vi "ReadVRMLog.vi"() -> (0 "time stamp":timestamp, 1 "X Field":dbl)   [LabVIEW 2013]
uses:
  <vilib>/Utility/file.llb/Read From Spreadsheet File (DBL).vi
  <vilib>/Utility/file.llb/Write To Spreadsheet File (DBL).vi
panel:
  in  "Tab Control":enum32{"Retrieved Log", "Storage"}(tab)
  out "XY Graph":cluster{timestamp[], dbl[]}(graph)
  out "XY Graph 2":cluster{"all rows":dbl[], "all rows":dbl[]}(graph)
  out "Set Points":dbl[][](graph)
  out "Magnet":dbl[][](graph)
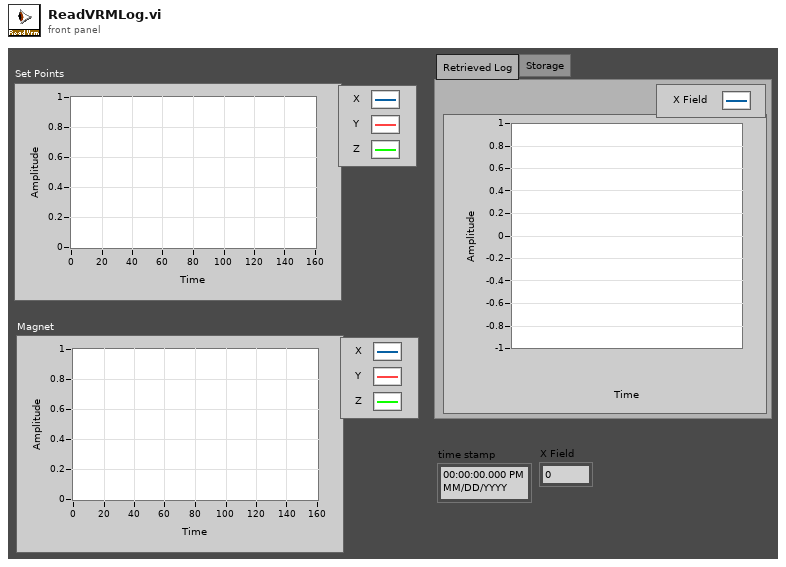
[diagram p1: front panel]
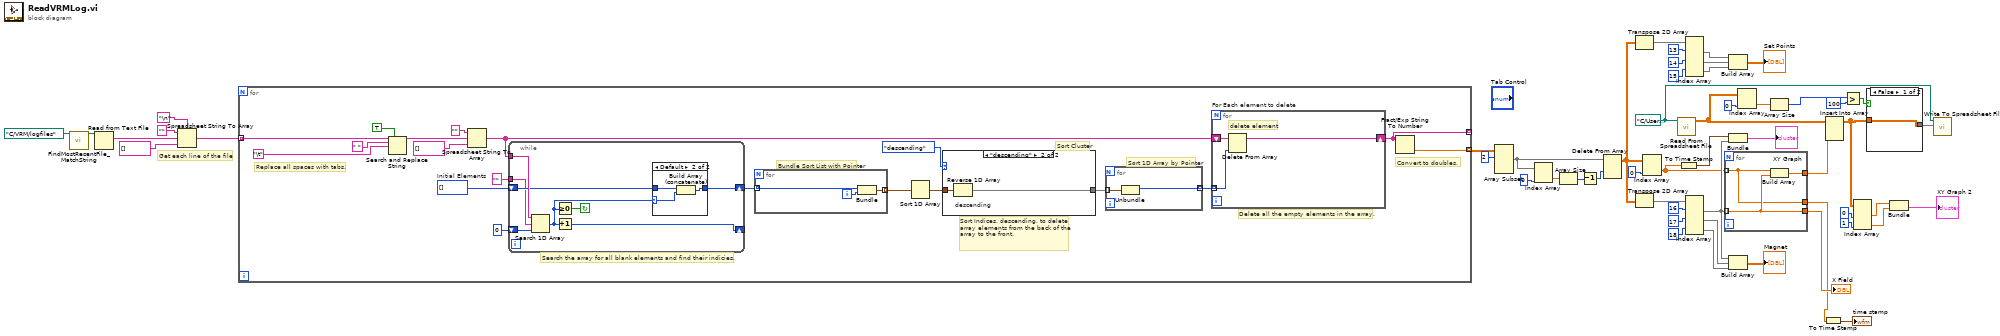
[diagram p0: block diagram]
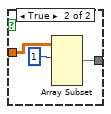
[diagram p2: hidden frame]
diagram:
  w23 = path "C:/Users/Voodoo/Desktop/Yun-Yi Pai/20140711 Log 2/Storage.txt" ("file path (dialog if empty)")
  # "Get each line of the file"
  n1 = call "FindMostRecentFile_MatchString.vi"("Folder Path In"=path "C:/VRM/logfiles") -> ("File Path Out"=w11:path)  [unwired: 9 in, 1 out]
  n2 = Read from Text File(file (use dialog)=w11) -> (text=w53:string)  [unwired: 1 in, 5 out]
  n3 = Spreadsheet String To Array(delimiter (Tab)="\n", format string="", spreadsheet string=w53, array type (2D Dbl)=string[] []) -> (array=w49:string[])
  n4 = for {
    tunnel: w49 -> [w72] mode=indexing
    tunnel: [w54] -> _ mode=indexing
    tunnel: [w55] -> w19 mode=indexing
    w64 = i32[] []  # Initial Elements
    # "Convert to doubles."
    # "Delete all the empty elements in the array."
    # "Search the array for all blank elements and find their indicies."
    # "Replace all spaces with tabs."
    # "Sort 1D Array by Pointer"
    # "Sort Cluster"
    # "Bundle Sort List with Pointer"
    # "Sort Indices, descending, to delete array elements from the back of the array to the front."
    n5 = Search and Replace String(replace all?=TRUE ("replace all? (F)"), input string=w72, search string=" ", replace string="\t") -> (result string=w67:string)  [unwired: 1 in, 6 out]
    n6 = Spreadsheet String To Array(format string="", spreadsheet string=w67, array type (2D Dbl)=string[] []) -> (array=w62:string[])  [unwired: 1 out]
    n7 = while {
      shift-right: [w84] -> _
      shift-left: 0 -> [w91]
      shift-right: [w88] -> w58
      shift-left: w64 -> [w89]
      tunnel: w62 -> [w90]
      tunnel: "" ("Element Data") -> [w87]
      stop <- w85 continue-if-true
      n8 = Search 1D Array(1D array=w90, element=w87, start index (0)=w91) -> (index of element=w86:i32)
      n9 = Greater Or Equal To 0?(x=w86) -> (x >= 0?=w85:bool)
      n10 = Increment(x=w86) -> (x+1=w84:i32)
      n11 = case shown="Default" w86 {
        selector: w86 -> [_ w95]
        tunnel: w89 -> [w92 w94]
        tunnel: [w92 w93] -> w88
        frame -1 {
        }
        frame Default {
          n12 = Build Array (concatenate)(w94, w95) -> (w93:i32[])
        }
      }
    }
    n13 = for {
      tunnel: w58 -> [w75] mode=indexing
      tunnel: [w73] -> w60 mode=indexing
      i -> [w74]
      n14 = Bundle("index of element"=w75, w74) -> (w73:cluster{"index of element":i32, i32})  [unwired: 1 out]
    }
    n15 = Sort 1D Array(array=w60) -> (sorted array=w59:cluster{"index of element":i32, i32}[])
    n16 = case shown="\"descending\"" enum16{"ascending", "descending"}."descending" ("Order") {
      tunnel: [w76 w77] -> w61
      tunnel: w59 -> [w76 w78]
      frame "ascending", Default {
      }
      frame "descending" {
        # "descending"
        n17 = Reverse 1D Array(array=w78) -> (reversed array=w77:cluster{"index of element":i32, i32}[])
      }
    }
    n18 = for {
      tunnel: w61 -> [w80] mode=indexing
      tunnel: [w79] -> w56 mode=indexing
      n19 = Unbundle(w80) -> ("index of element"=w79:i32)  [unwired: 1 out]
    }
    n20 = for "For Each element to delete" {
      tunnel: w56 -> [w83] mode=indexing
      shift-right: [w82] -> w54
      shift-left: w62 -> [w81]
      # "delete element"
      n21 = Delete From Array(array=w81, index=w83) -> (array with subset deleted=w82:string[])  [unwired: 1 in, 1 out]
    }
    n22 = Fract/Exp String To Number(string=w54) -> (number=w55:dbl[])  [unwired: 4 out]
  }
  n23 = Array Subset(array=w19, index (row)=2 ("index")) -> (w13:dbl[][])  [unwired: 3 in]
  n24 = Index Array(array=w13, index (col)=0 ("disabled index (col)")) -> (element=w17:dbl[])  [unwired: 1 in]
  n25 = Array Size(array=w17) -> (size(s)=w15:i32)
  n26 = Decrement(x=w15) -> (x-1=w14:i32)
  n27 = Delete From Array(array=w13, index (row)=w14) -> (array with subset deleted=w16:dbl[][])  [unwired: 2 in, 1 out]
  n28 = Transpose 2D Array(2D array=w16) -> (transposed array=w48:dbl[][])
  n29 = Transpose 2D Array(2D array=w16) -> (transposed array=w37:dbl[][])
  n30 = Index Array(array=w16, index (col)=0 ("index (row)")) -> (element=w20:dbl[])  [unwired: 1 in]
  n31 = call-poly <vilib>:"Read From Spreadsheet File.vi"("file path (dialog if empty)"=w23) -> ("all rows"=w27:dbl[][])  [unwired: 6 in, 4 out]
  n32 = To Time Stamp(1:w20) -> (0:w31:timestamp[])
  n33 = Index Array(array=w48, index (row) #1=13 ("index (row)"), index (row) #2=14 ("index (row)"), index (row) #3=15 ("index (row)")) -> (element #1=w35:dbl[], element #2=w34:dbl[], element #3=w33:dbl[])  [unwired: 3 in]
  n34 = Index Array(array=w37, index (row) #1=16 ("index (row)"), index (row) #2=17 ("index (row)"), index (row) #3=18 ("index (row)")) -> (element #1=w30:dbl[], element #2=w40:dbl[], element #3=w39:dbl[])  [unwired: 3 in]
  n35 = for {
    tunnel: w30 -> [w97] mode=indexing
    tunnel: w20 -> [w96] mode=indexing
    tunnel: [w98] -> w21
    tunnel: [w97] -> w3
    tunnel: [w96] -> w2
    n36 = Build Array(w96, w97) -> (w98:dbl[])
  }
  "X Field" <- w3
  n37 = Build Array(w35, w34, w33) -> (→"Set Points":dbl[][])
  n38 = Bundle(w31, w30) -> (→"XY Graph":cluster{timestamp[], dbl[]})  [unwired: 1 in]
  n39 = Build Array(w30, w40, w39) -> (→"Magnet":dbl[][])
  n40 = Index Array(array=w27, index (col)=0 ("index (row)")) -> (element=w29:dbl[])  [unwired: 1 in]
  n41 = Array Size(array=w29) -> (size(s)=w26:i32)
  n42 = To Time Stamp(1:w2) -> (0:→"time stamp":timestamp)
  n43 = Insert Into Array(array=w27, new element=w21) -> (w9:dbl[][])  [unwired: 2 in]
  n44 = Greater?(x=w26, y=100) -> (0:w24:bool)
  n45 = Index Array(array=w9, index (col) #1=0 ("index (row)"), index (col) #2=1 ("index (row)")) -> (element #1=w8:dbl[], element #2=w7:dbl[])  [unwired: 2 in]
  n46 = case shown="False" w24 {
    tunnel: w9 -> [w99 w102]
    tunnel: [w99 w100] -> w22
    frame False {
    }
    frame True {
      n47 = Array Subset(array=w102, index (row)=1 ("index")) -> (w100:dbl[][])  [unwired: 3 in]
    }
  }
  n48 = Bundle("all rows"=w8, "all rows"=w7) -> (→"XY Graph 2":cluster{"all rows":dbl[], "all rows":dbl[]})  [unwired: 1 in]
  n49 = call-poly <vilib>:"Write To Spreadsheet File.vi"("2D data"=w22, "file path (dialog if empty)"=w23) -> ()  [unwired: 6 in, 1 out]
